vi "Bucket Similar Diff Images.vi"(6 "match threshold (.985)":dbl=0.985 format="%#_13g", 10 "All PNG Files":path[](array[path])) -> (3 "All PNG Files (Bucketed by Near-Matches)":cluster{"Similar PNG Files":path[]}[](array[cluster]))   [LabVIEW 2020, in "Graphical Diff.lvlib"]
uses:
  Graphical Diff.lvlib
panel:
  out "Image buckets":i32[](array[numeric])
  out "Report":string
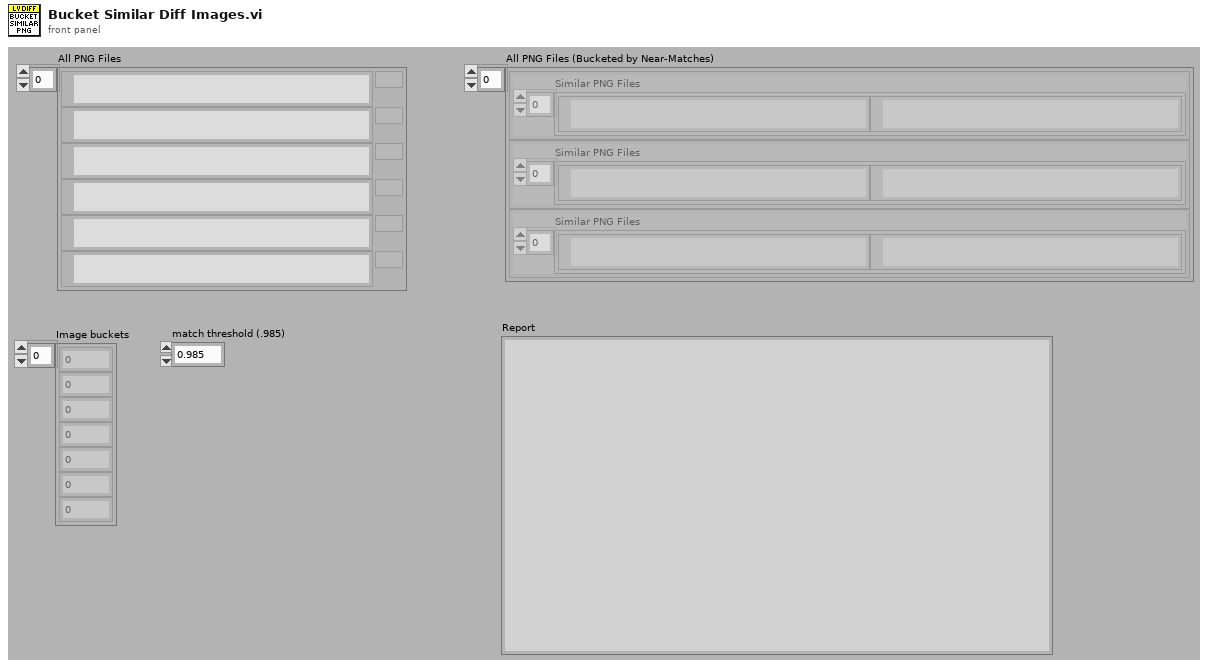
[diagram p1: front panel]
types:
  T1 = typedef "imagedata.ctl" = cluster{"image type":i32, "image depth":i32, "image":u8[], "mask":u8[], "colors":u32[], "Rectangle":cluster{"left":i16, "top":i16, "right":i16, "bottom":i16}}
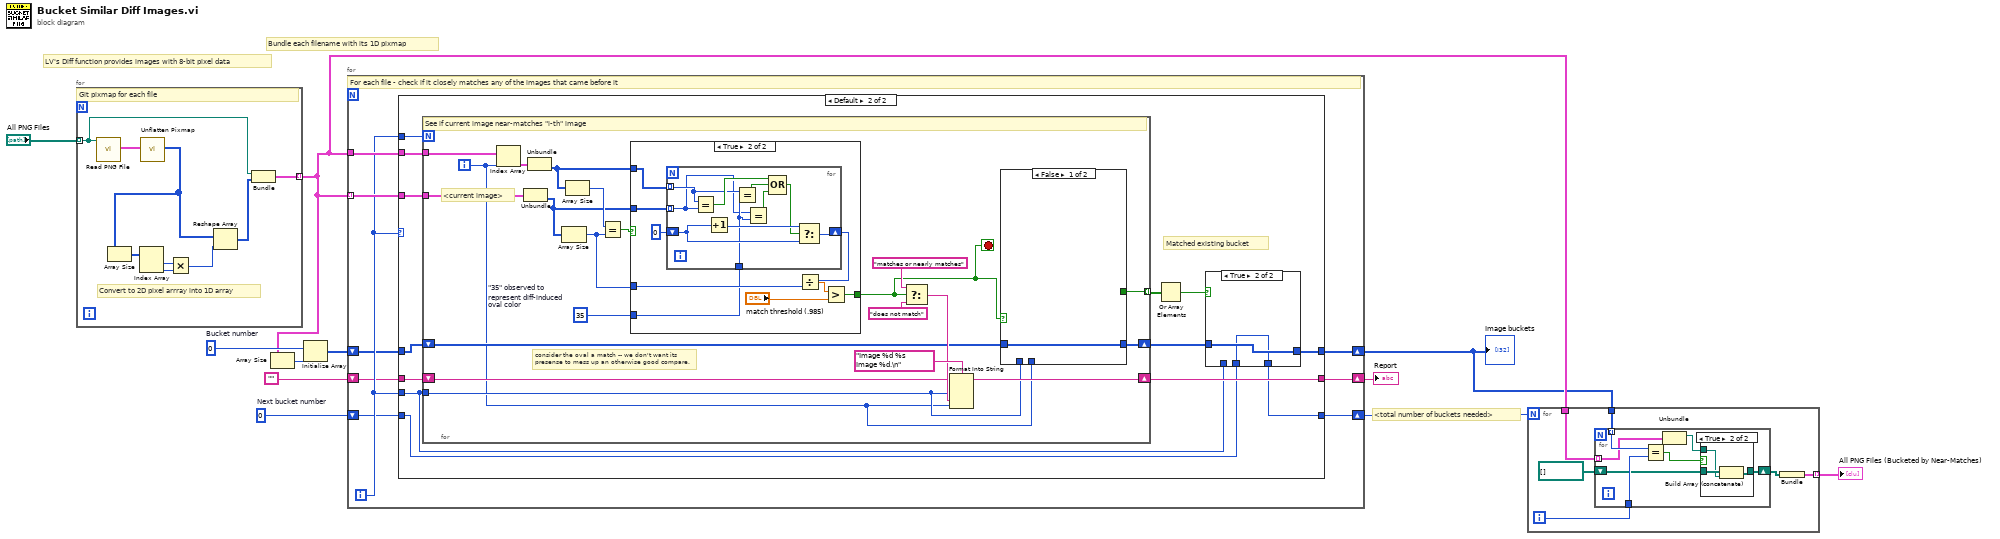
[diagram p0: block diagram]
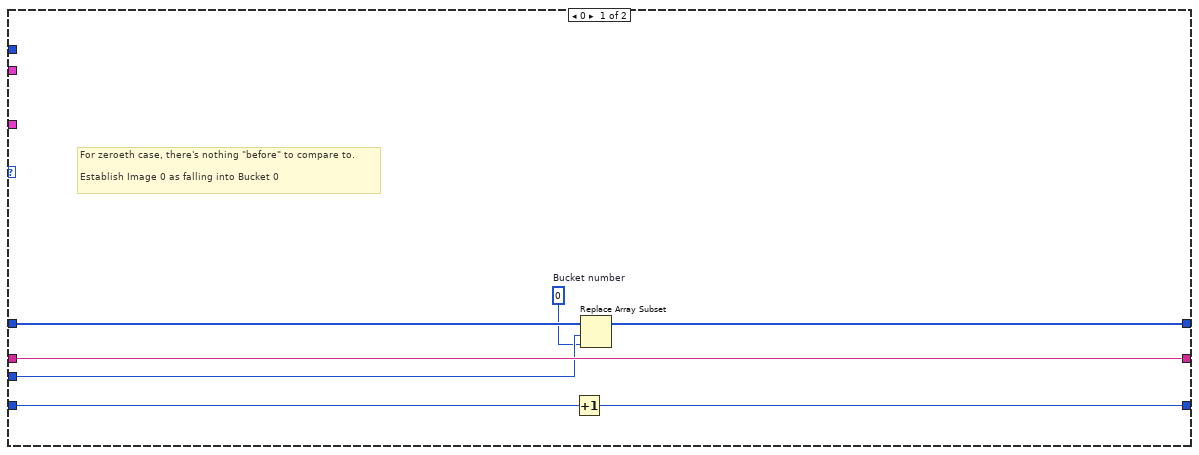
[diagram p3: hidden frame]
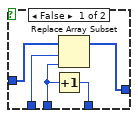
[diagram p4: hidden frame]
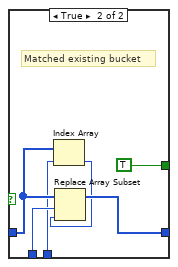
[diagram p5: hidden frame]
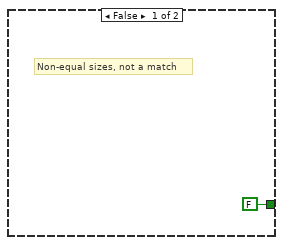
[diagram p6: hidden frame]
diagram:
  w5 = 0  # Next bucket number
  w8 = 0  # Bucket number
  # "<total number of buckets needed>"
  # "Bundle each filename with its 1D pixmap"
  # "LV's Diff function provides images with 8-bit pixel data"
  n1 = for {
    tunnel: "All PNG Files" -> [w14] mode=indexing
    tunnel: [w12] -> w3 mode=indexing
    # "Convert to 2D pixel arrray into 1D array"
    # "Git pixmap for each file"
    n2 = call <vilib>:"Read PNG File.vi"("path to PNG file"=w14) -> ("image data"=w20:T1)  [unwired: 8 in, 2 out]
    n3 = call <vilib>:"Unflatten Pixmap.vi"("image data"=w20) -> ("8-bit pixmap"=w15:u8[][])  [unwired: 4 in, 6 out]
    n4 = Array Size(array=w15) -> (size(s)=w19:i32[])
    n5 = Index Array(array=w19) -> (element #1=w17:i32, element #2=w18:i32)  [unwired: 2 in]
    n6 = Multiply(x=w17, y=w18) -> (x*y=w16:i32)
    n7 = Reshape Array(w15, w16) -> (w13:u8[])
    n8 = Bundle("Path"=w14, "8-bit pixmap"=w13) -> (w12:cluster{"Path":path, "8-bit pixmap":u8[]})  [unwired: 1 in]
  }
  n9 = Array Size(array=w3) -> (size(s)=w7:i32)
  n10 = Initialize Array(w8, w7) -> (w6:i32[])
  n11 = for {
    tunnel: w3 -> [w29] mode=indexing
    tunnel: w3 -> [w28]
    shift-right: [w25] -> w9
    shift-left: "" -> [w26]
    shift-right: [w23] -> w2
    shift-left: w6 -> [w24]
    shift-right: [w21] -> w4
    shift-left: w5 -> [w22]
    i -> [w27]
    # "For each file - check if it closely matches any of the images that came before it"
    n12 = case shown="Default" w27 {
      tunnel: w27 -> [_ w49]
      tunnel: w29 -> [_ w48]
      tunnel: w28 -> [_ w47]
      tunnel: w27 -> [w33 w37]
      tunnel: w26 -> [w36 w46]
      tunnel: [w36 w45] -> w25
      tunnel: w24 -> [w35 w44]
      tunnel: [w34 w41] -> w23
      tunnel: w22 -> [w31 w39]
      tunnel: [w30 w38] -> w21
      frame 0 {
        w32 = 0  # Bucket number
        # "For zeroeth case, there's nothing \"before\" to compare to.\n\nEstablish Image 0 as falling into Bucket 0"
        n13 = Increment(x=w31) -> (x+1=w30:i32)
        n14 = Replace Array Subset(array=w35, new element=w32, index=w33) -> (w34:i32[])
      }
      frame Default {
        # "Matched existing bucket"
        n15 = for {
          N: w49 -> [_]
          tunnel: w48 -> [w75]
          tunnel: w47 -> [w77]
          tunnel: w37 -> [w60]
          shift-right: [w64] -> w45
          shift-left: w46 -> [w65]
          shift-right: [w61] -> w40
          shift-left: w44 -> [w62]
          tunnel: [w58] -> w43 mode=indexing
          i -> [w59]
          stop <- w63 stop-if-true
          w57 = u8 35  # "35" observed to represent diff-induced oval color
          # "consider the oval a match -- we don't want its presense to mess up an otherwise good compare."
          # "<current image>"
          # "See if current image near-matches \"i-th\" image"
          n16 = Index Array(array=w77, index=w59) -> (element=w76:cluster{"Path":path, "8-bit pixmap":u8[]})
          n17 = Unbundle(w75) -> ("8-bit pixmap"=w71:u8[])  [unwired: 1 out]
          n18 = Unbundle(w76) -> ("8-bit pixmap"=w72:u8[])  [unwired: 1 out]
          n19 = Array Size(array=w71) -> (size(s)=w70:i32)
          n20 = Array Size(array=w72) -> (size(s)=w74:i32)
          n21 = Equal?(x=w74, y=w70) -> (x = y?=w73:bool)
          n22 = case shown="True" w73 {
            tunnel: w72 -> [_ w94]
            tunnel: w71 -> [_ w93]
            tunnel: w70 -> [_ w91]
            tunnel: [FALSE w87] -> w63
            tunnel: w57 -> [_ w86]
            frame False {
              # "Non-equal sizes, not a match"
            }
            frame True {
              n23 = for {
                tunnel: w94 -> [w99] mode=indexing
                tunnel: w93 -> [w95] mode=indexing
                shift-right: [w104] -> w90
                shift-left: 0 -> [w102]
                tunnel: w86 -> [w96]
                n24 = Equal?(x=w99, y=w95) -> (x = y?=w101:bool)
                n25 = Increment(x=w102) -> (x+1=w103:i32)
                n26 = Equal?(x=w99, y=w96) -> (x = y?=w98:bool)
                n27 = Equal?(x=w95, y=w96) -> (x = y?=w97:bool)
                n28 = Compound Arithmetic op=OR(w101, w98, w97) -> (w100:bool)
                n29 = Select(t=w103, s=w100, f=w102) -> (s? t:f=w104:i32)
              }
              n30 = Divide(x=w90, y=w91) -> (x/y=w89:dbl)
              n31 = Greater?(x=w89, y="match threshold (.985)") -> (0:w87:bool)
            }
          }
          n32 = Select(t="matches or nearly matches", s=w63, f="does not match") -> (s? t:f=w66:string)
          n33 = Format Into String(format string="Image %d %s Image %d.\n", initial string=w65, w60, w66, w59) -> (resulting string=w64:string)  [unwired: 1 in, 1 out]
          n34 = case shown="False" w63 {
            tunnel: w62 -> [w78 w82]
            tunnel: [w78 w84] -> w61
            tunnel: w60 -> [_ w83]
            tunnel: w59 -> [_ w81]
            tunnel: [_ TRUE] -> w58
            frame False {
            }
            frame True {
              # "Matched existing bucket"
              n35 = Index Array(array=w82, index=w81) -> (element=w80:i32)
              n36 = Replace Array Subset(array=w82, new element=w80, index=w83) -> (w84:i32[])
            }
          }
        }
        n37 = Or Array Elements(Boolean array=w43) -> (logical OR=w42:bool)
        n38 = case shown="True" w42 {
          tunnel: [w53 w56] -> w41
          tunnel: w40 -> [w54 w56]
          tunnel: w39 -> [w51 w55]
          tunnel: [w50 w55] -> w38
          tunnel: w37 -> [w52 _]
          frame False {
            n39 = Increment(x=w51) -> (x+1=w50:i32)
            n40 = Replace Array Subset(array=w54, new element=w51, index=w52) -> (w53:i32[])
          }
          frame True {
          }
        }
      }
    }
  }
  "Report" <- w9
  "Image buckets" <- w2
  n41 = for {
    N: w4 -> [_]
    tunnel: w3 -> [w110]
    tunnel: w2 -> [w109]
    tunnel: [w105] -> w1 mode=indexing
    i -> [w108]
    n42 = for {
      tunnel: w110 -> [w115] mode=indexing
      tunnel: w109 -> [w116] mode=indexing
      tunnel: w108 -> [w117]
      shift-right: [w112] -> w106
      shift-left: path[] [] ("Similar PNG Files") -> [w111]
      n43 = Equal?(x=w116, y=w117) -> (x = y?=w114:bool)
      n44 = Unbundle(w115) -> ("Path"=w113:path)  [unwired: 1 out]
      n45 = case shown="True" w114 {
        tunnel: w113 -> [_ w120]
        tunnel: [w118 w119] -> w112
        tunnel: w111 -> [w118 w121]
        frame False {
        }
        frame True {
          n46 = Build Array (concatenate)(w121, w120) -> (w119:path[])
        }
      }
    }
    n47 = Bundle("Similar PNG Files"=w106) -> (w105:cluster{"Similar PNG Files":path[]})  [unwired: 1 in]
  }
  "All PNG Files (Bucketed by Near-Matches)" <- w1
